vi "Actor Core.vi"(8 "error in":errorcluster, 11 "uService Template in":refnum<class "Common GUI v3.lvclass">) -> (0 "error out":errorcluster, 3 "Actor out":refnum<class "Actor.lvclass">)   [LabVIEW 2026, in "TALOS.lvlib" / "Common GUI v3.lvlib" / "Common GUI v3.lvclass"]
doc: "(<B>Filename</B>: Actor Framework.lvlib:Actor.lvclass:Actor Core.vi)\n\nReceives messages to the actor, reacts to them, and initiates any error handling that may shut the actor down.\n\nDescendant classes may override this VI to append parallel tasks for the actor to complete while it handles messages. Overrides use the Call Parent Class Method node."
uses:
  Common GUI v3.lvclass
  C:/LabVIEW Code/TALOS/builds/Actor Framework PPL/Actor Framework.lvlibp/1abvi3w/vi.lib/ActorFramework/Actor/Actor.lvclass
  C:/LabVIEW Code/TALOS/talos/Father of all uServices/Father of all uServices/Father of all uServices.lvclass
  builds/Actor Framework PPL/Actor Framework.lvlibp/1abvi3w/vi.lib/ActorFramework/Actor/Actor.lvclass
  Common GUI v3.lvclass/Common GUI v3.ctl
  Classes/uService List/uService List.lvclass/uService List.ctl
  Ancestor/Ancestor/Ancestor.lvclass/Ancestor.ctl
  Guardian/Guardian/Buttons_UI.ctl
  Guardian/Guardian Messages/Button Pressed Msg/Button Pressed Msg.lvclass/Button Pressed Msg.ctl
  Remote uService GUI.ctl
  Common GUI v3 Consumer Case Selector.ctl
  Father of all uServices/Father of all uServices Messages/Consumer Msg/Consumer Msg.lvclass/Consumer Msg.ctl
  builds/Actor Framework PPL/Actor Framework.lvlibp/1abvi3w/vi.lib/ActorFramework/Message Enqueuer/Message Priority.ctl
  Ancestor/Ancestor Messages/Process EH Error Msg/Process EH Error Msg.lvclass/Process EH Error Msg.ctl
  Classes/uService List/Get VI Ref.vi
  Classes/uService List/Get Remote GUI.vi
  Classes/uService List/Get Remote Window VI Ref.vi
  Classes/uService List/Get all IDs.vi
  Classes/uService List/Get Properties.vi
  Support VIs/Generate Error.vi
  Father of all uServices/Father of all uServices Messages/Consumer Msg/Send Consumer.vi
  FGV/Error Memory/Get Error Description.vi
  Support VIs/Get PC name.vi
  Ancestor/Ancestor/Read ID.vi
  Support VIs/Get Class Name.vi
  FGV/Error Memory/Error Memory Core.vi
  <vilib>/AdvancedString/Delimited String to 1D String Array.vi
  <vilib>/AdvancedString/Delimited String to 1D String Array (string).vi
  Support VIs/Circus Root Path.vi
  FGV/Error Memory/Error Crt Lvl checker.vi
  FGV/Error Memory/Error Memory Core.vi/40c8088d-b597-4017-91af-faa98e00292e.vi
  FGV/Error Memory/Error Memory Core.vi/d4a3ab98-063c-4e44-b43d-fbdcfe6c2be2.vi
  Father of all uServices/Father of all uServices/Father of all uServices.lvclass
  Support VIs/Global Memory.vi
  <vilib>/Utility/LVClass/Get LV Class Name.vi
  Support VIs/Is in Packed Library.vi
  Support VIs/TALOS Root path.vi
  Support VIs/Read CSV worksheet.vi
  Support VIs/Global Constants.vi
  <vilib>/Utility/error.llb/General Error Handler.vi
  Support VIs/Error Log.vi
  builds/Actor Framework PPL/Actor Framework.lvlibp/1abvi3w/vi.lib/ActorFramework/Message Enqueuer/Enqueue.vi
  <userlib>/_OpenG.lib/lvdata/lvdata.llb/Get Strings from Enum__ogtk.vi
  builds/Actor Framework PPL/Actor Framework.lvlibp/1abvi3w/vi.lib/ActorFramework/Message Enqueuer/Message Enqueuer.lvclass
  Ancestor/Ancestor/Ancestor.lvclass
  <vilib>/Comparison/Equal/Equal Functor/Equal Functor.lvclass
  Guardian/Guardian Messages/Button Pressed Msg/Button Pressed Msg.lvclass
  Father of all uServices/Father of all uServices Messages/Consumer Msg/Consumer Msg.lvclass
  Ancestor/Ancestor Messages/Process EH Error Msg/Process EH Error Msg.lvclass
  Guardian/Guardian/Guardian.lvclass
  Classes/uService List/uService List.lvclass
  TALOS.lvlib
  Common GUI v3.lvlib
panel:
  in  "stop":bool
  in  "remote GUI":bool
  out "Circus Logo":picture
  in  "All uS":bool
  out "Errors":i32(listbox)
  out "uServices Online":T1(c390)
  out "Guardians List":T1(c390)
  out "Run Configuration":string
  out "Run Number":u32
  out "Error Details":string
  out "Kasli Log":string
  out "RUN":bool
  in  "uService to show":string(combo)
  out "ABORT":bool
  out "Guardian ID":string
  # "PRESS CTRL TO ARM"
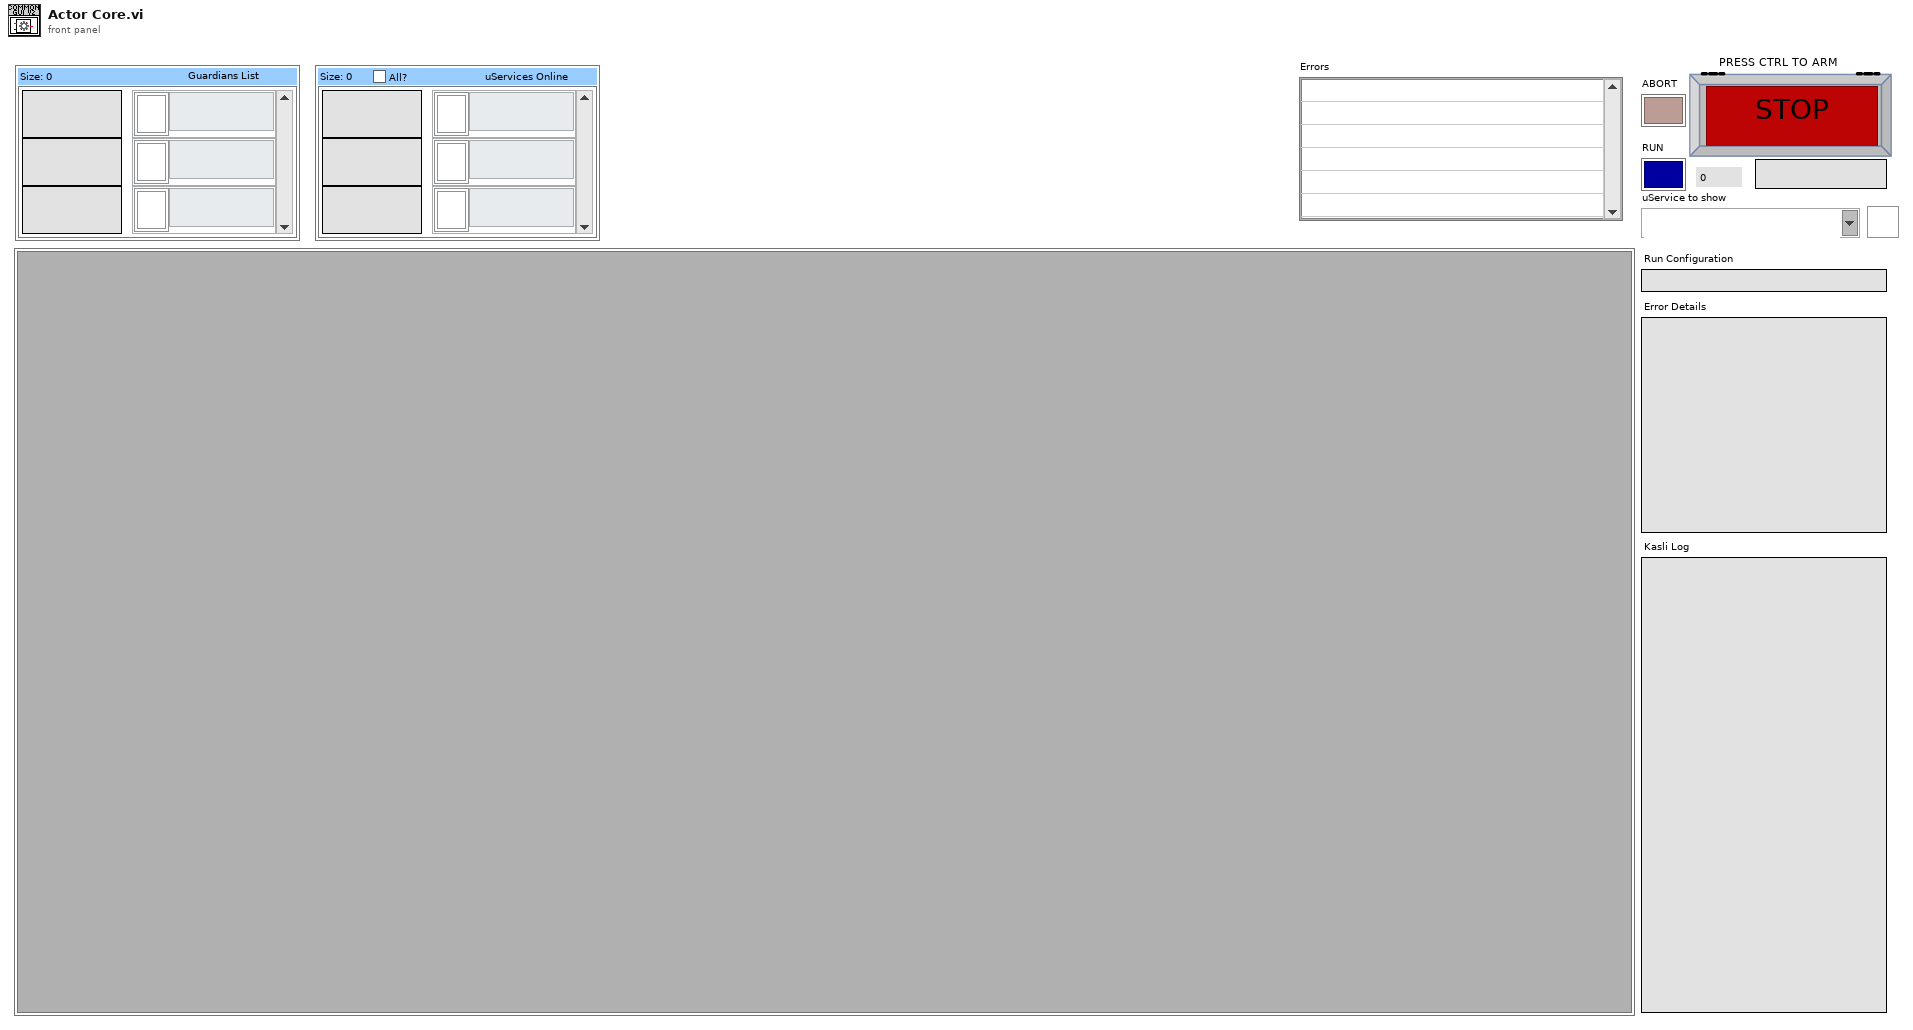
[diagram p1: front panel]
types:
  T1 = map{string, cluster{"Online":bool, "Last Pat":timestamp}}
  T2 = enum16{"None", "On Hover", "On Key Focus", "On Hover or Key Focus"}
  T3 = typedef "TALOS.lvlib/Guardian.lvlib/Guardian.lvclass/Buttons_UI.ctl" = enum16{"Start uService", "Kill uService", "Stop uService", "Stop", "Start online checks", "Stop online checks", "Send Pat to all GDs", "Reload INI files", "Update from GIT", "RUN", "Reset ABORT", "Check Bearer", "Send I Exist", "Change Run Config", "Add uSs from Config", "Realign uSs from Config", "Send Run Config to GD"}
  T4 = typedef "TALOS.lvlib/Common GUI v3.lvlib/Common GUI v3.lvclass/Common GUI v3 Consumer Case Selector.ctl" = enum16{"Update Guardians List", "Update ABORT LED", "Update Guardian ID", "Update Kasli Log", "Update Error Listbox", "Update Run Number", "Change Run LED color", "Update Run Status", "Run Stopped with Errors", "Reset Run LED", "Update Run Config", "Remote GUI"}
  T5 = typedef "TALOS.lvlib/Common GUI v3.lvlib/Remote uService GUI.ctl" = cluster{"Open/Close":bool, "uService ID":string}
  T6 = typedef "Actor Framework.lvlibp/Message Enqueuer.lvclass/Message Priority.ctl" = enum16{"Low", "Normal", "High"}
  T7 = typedef "lveventtype.ctl" = enum32{"Null", "Timeout", "Annotation Menu Selection", "Annotation Menu Selection?", "App Instance Close", "App Instance Close?", "Autoscale Range Change", "Bookmark Info Change", "Cell Edit", "Cell Edit?", "Cursor Grab", "Cursor Grab?", "Cursor Menu Selection", "Cursor Menu Selection?", "Cursor Move", "Cursor Release", "Data Change", "Direction Change", "Display State Change", "Drag Ended", "Drag Enter", "Drag Leave", "Drag Over", "Drag Source Update", "Drag Starting", "Drag Starting?", "Drop", "Exec State Change", "Key Down", "Key Down?", "Key Repeat", "Key Repeat?", "Key Up", "Listbox Double Click", "Menu Activation?", "Menu Selection (App)", "Menu Selection? (App)", "Menu Selection (User)", "Mouse Down", "Mouse Down?", "Mouse Enter", "Mouse Leave", "Mouse Move", "Mouse Up", "Mouse Wheel", "NI Security User Change (App)", "Pane Size", "Panel Close", "Panel Close?", "Panel Resize", "Plot Attribute Change", "Scale Range Change", "Shortcut Menu Activation?", "Shortcut Menu Selection (App)", "Shortcut Menu Selection? (App)", "Shortcut Menu Selection (User)", "Tree Double Click", "Tree Drag", "Tree Drag?", "Tree Drop", "Tree Drop?", "Tree Item Close", "Tree Item Close?", "Tree Item Open", "Tree Item Open?", "URL Change?", "User Event", "Value Change"}
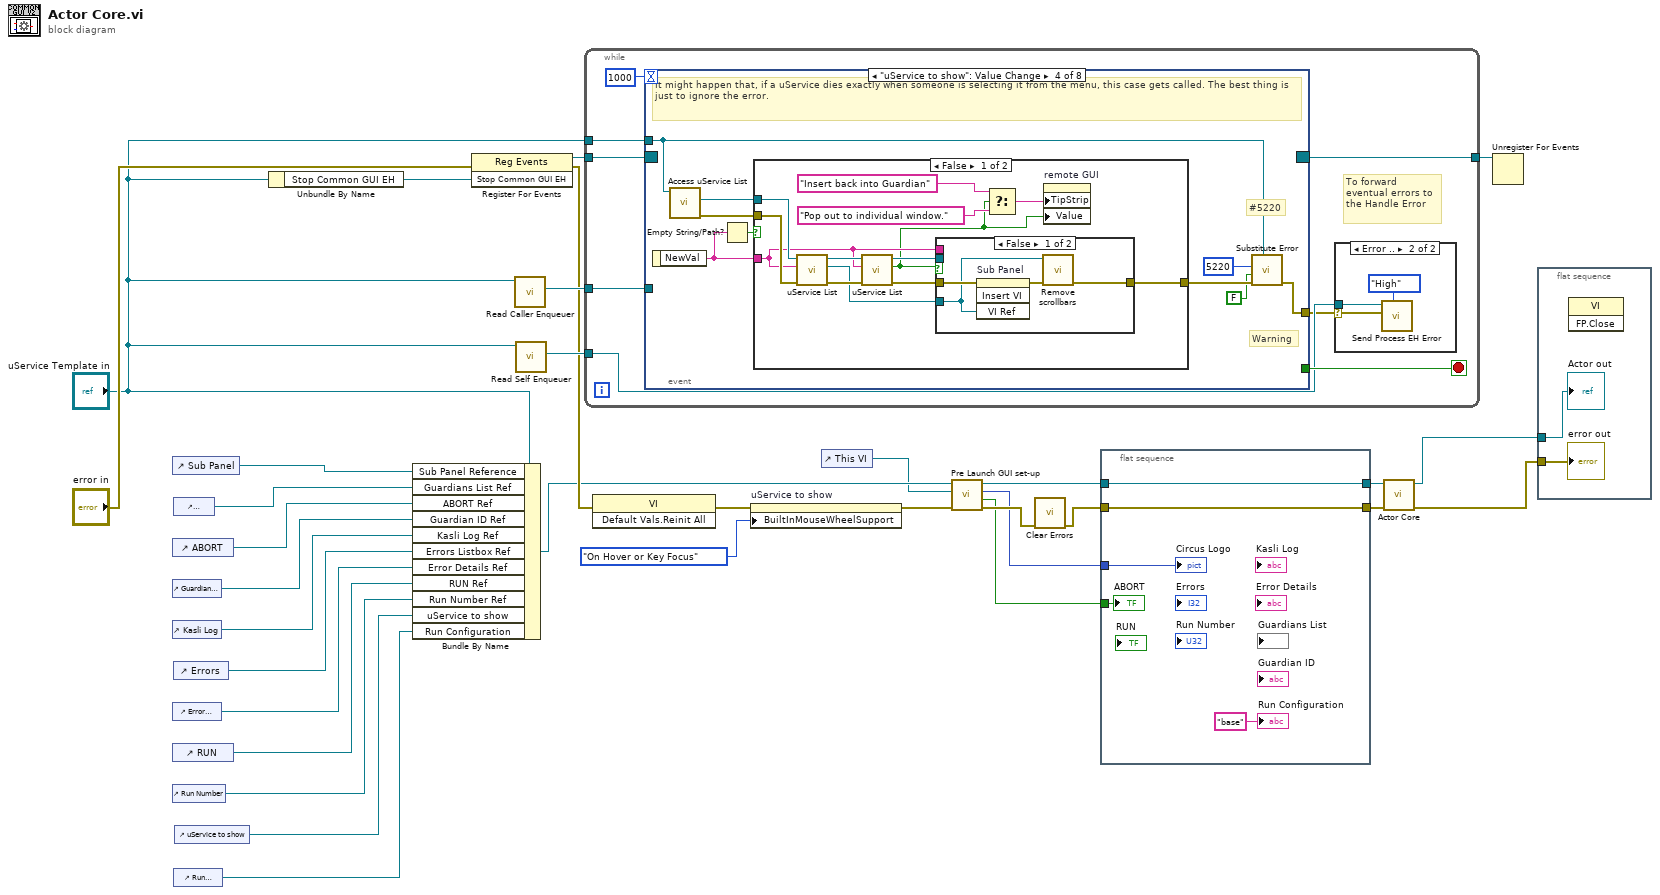
[diagram p0: block diagram]
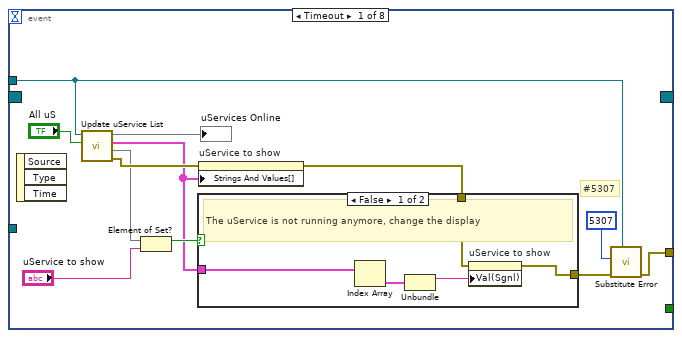
[diagram p2: hidden frame]
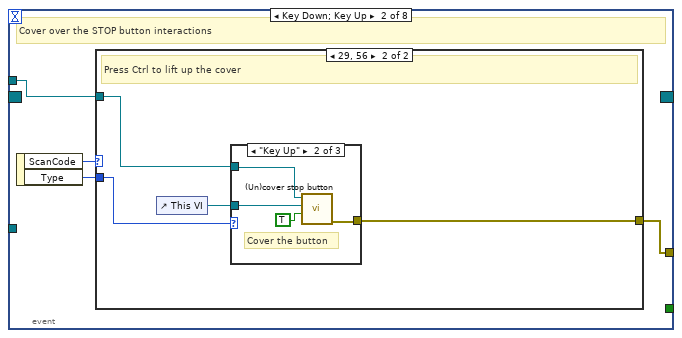
[diagram p4: hidden frame]
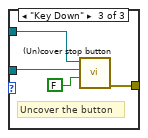
[diagram p7: hidden frame]
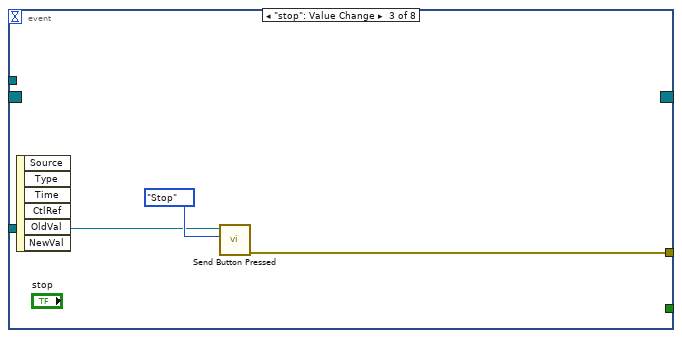
[diagram p8: hidden frame]
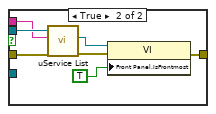
[diagram p9: hidden frame]
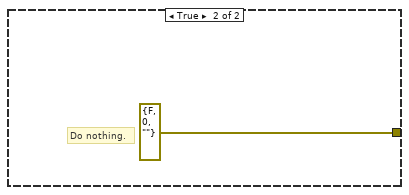
[diagram p10: hidden frame]
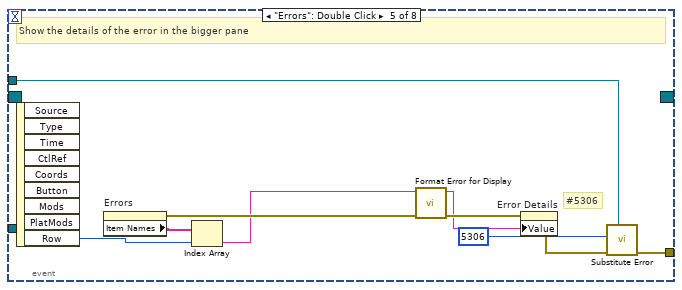
[diagram p11: hidden frame]
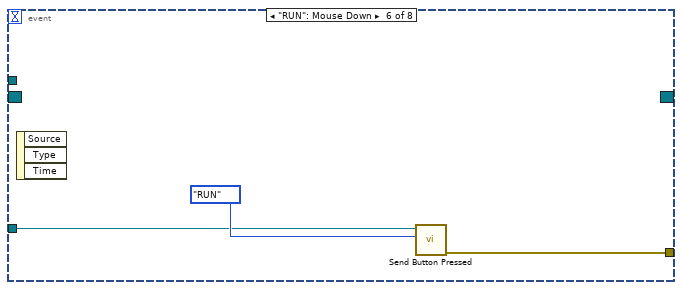
[diagram p12: hidden frame]
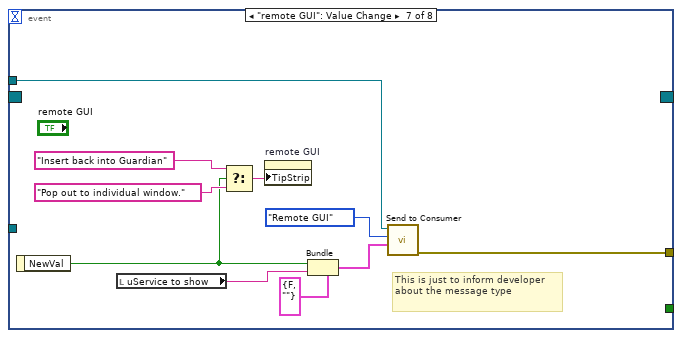
[diagram p13: hidden frame]
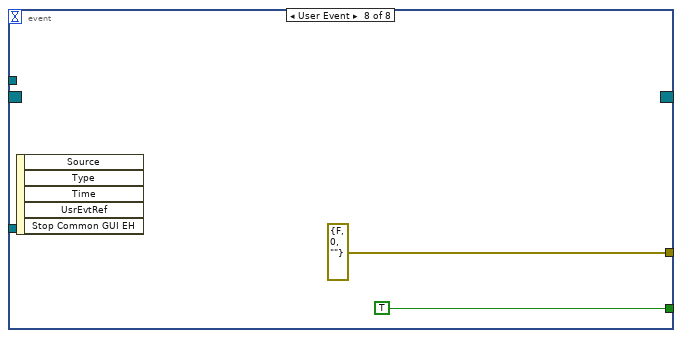
[diagram p14: hidden frame]
diagram:
  n1 = control-ref of="Sub Panel"() -> (w29:refnum<vi>)
  n2 = control-ref of="ABORT"() -> (w22:refnum<vi>)
  n3 = control-ref of="Guardian ID"() -> (w21:refnum<vi>)
  n4 = control-ref of="Kasli Log"() -> (w20:refnum<vi>)
  n5 = control-ref of="Error Details"() -> (w18:refnum<vi>)
  n6 = control-ref of="RUN"() -> (w16:refnum<vi>)
  n7 = control-ref of="Run Number"() -> (w15:refnum<vi>)
  n8 = control-ref of="Guardians List"() -> (w23:refnum<vi>)
  n9 = control-ref of="Errors"() -> (w19:refnum<vi>)
  n10 = control-ref of="Run Configuration"() -> (w5:refnum<vi>)
  n11 = control-ref of="uService to show"() -> (w12:refnum<vi>)
  n12 = Unbundle By Name("uService Template in") -> ("Stop Common GUI EH"=w28:refnum<user-event>)
  n13 = Bundle By Name(cluster="uService Template in", "Sub Panel Reference"=w29, "Guardians List Ref"=w23, "ABORT Ref"=w22, "Guardian ID Ref"=w21, "Kasli Log Ref"=w20, "Errors Listbox Ref"=w19, "Error Details Ref"=w18, "RUN Ref"=w16, "Run Number Ref"=w15, "uService to show"=w12, "Run Configuration"=w5) -> (w11:refnum<class "Common GUI v3.lvclass">)
  n14 = register-events(error in="error in", w28) -> (reference out=w27:refnum<event-registration>, error out=w17:errorcluster)  [unwired: 1 in]
  n15 = call "Read Caller Enqueuer.vi"("Actor"="uService Template in") -> ("Caller Enqueuer"=w25:refnum<class "Message Enqueuer.lvclass">)  [unwired: 10 in]
  n16 = call "Read Self Enqueuer.vi"("Actor"="uService Template in") -> ("Self Enqueuer"=w24:refnum<class "Message Enqueuer.lvclass">)  [unwired: 10 in]
  n17 = while {
    tunnel: w27 -> [w41]
    tunnel: [w39] -> w26
    tunnel: w25 -> [w38]
    tunnel: w24 -> [w36]
    tunnel: "uService Template in" -> [w34]
    stop <- w40 stop-if-true
    # "To forward eventual errors to the Handle Error"
    n18 = event shown="[3] \"uService to show\": Value Change" {
      selector: w41 -> [_ _ _ _ _ _ _ _]
      dyn-events: [_ _ _ _ _ _ _ _] -> w39
      timeout: 1000 -> [_ _ _ _ _ _ _ _]
      tunnel: [_ _ _ _ _ _ _ TRUE] -> w40
      tunnel: w38 -> [_ _ w77 _ _ w124 _ _]
      tunnel: [w45 w60 w76 w84 w119 w123 w132 errorcluster {"status"=FALSE, "code"=0, "source"=""} ("error out")] -> w35
      tunnel: w34 -> [w44 w61 _ w81 w118 _ w131 _]
      event Timeout {
        # "#5307"
        n19 = event-data() -> ()  [unwired: 1 in, 3 out]
        n20 = call "Update uService List.vi"("All uS?"="All uS", "Common GUI v3 in"=w44) -> ("error out"=w53:errorcluster, "Check currently displayed"=w51:set{string}, "For ComboBox"=w48:cluster{"ID":string, "ID":string}[], "Map"=→"uServices Online":map{string, cluster{bool, "Last Pat":timestamp}})  [unwired: 5 in, 1 out]
        n21 = Element of Set?(10:"uService to show", 11:w51) -> (3:w49:bool)
        n22 = property on="uService to show" class="CmbBox"(error in=w53, "Strings And Values[]"=w48) -> (error out=w47:errorcluster)  [unwired: 1 in, 1 out]
        n23 = case shown="False" w49 {
          tunnel: w48 -> [w58 _]
          tunnel: w47 -> [w55 w59]
          tunnel: [w54 w59] -> w46
          frame False {
            # "The uService is not running anymore, change the display"
            n24 = Index Array(array=w58) -> (element=w57:cluster{"ID":string, "ID":string})  [unwired: 1 in]
            n25 = Unbundle(w57) -> ("ID"=w56:string)  [unwired: 1 out]
            n26 = property on="uService to show" class="CmbBox"(error in=w55, "Val(Sgnl)"=w56) -> (error out=w54:errorcluster)  [unwired: 1 in, 1 out]
          }
          frame True {
            # "It's still present, OK"
          }
        }
        n27 = call "Substitute Error.vi"("LabVIEW Object"=w44, "error in (no error)"=w46, "Error Code"=5307) -> ("error out"=w45:errorcluster)  [unwired: 8 in]
      }
      event Key Down; Key Up {
        # "Cover over the STOP button interactions"
        n28 = event-data() -> ("ScanCode"=w63:i16, "Type"=w62:T7)  [unwired: 1 in]
        n29 = case shown="29, 56" w63 {
          tunnel: w62 -> [_ w67]
          tunnel: w61 -> [_ w65]
          tunnel: [_ w64] -> w60
          frame Default {
            # "Any other button, do nothing"
          }
          frame 29, 56 {
            # "Press Ctrl to lift up the cover"
            n30 = control-ref of="This VI"() -> (w66:refnum<vi>)
            n31 = case shown="\"Key Up\"" w67 {
              tunnel: [_ w68 w75] -> w64
              tunnel: w66 -> [_ w70 w73]
              tunnel: w65 -> [_ w69 w72]
              frame "Null", Default {
              }
              frame "Key Up" {
                # "Cover the button"
                n32 = call-dynamic "(Un)cover stop button.vi"("Cover/Uncover"=TRUE, "GUI ref in"=w70, "Common GUI v3 in"=w69) -> ("error out"=w68:errorcluster)  [unwired: 6 in, 2 out]
              }
              frame "Key Down" {
                # "Uncover the button"
                n33 = call-dynamic "(Un)cover stop button.vi"("Cover/Uncover"=FALSE, "GUI ref in"=w73, "Common GUI v3 in"=w72) -> ("error out"=w75:errorcluster)  [unwired: 6 in, 2 out]
              }
            }
          }
        }
      }
      event "stop": Value Change {
        n34 = event-data() -> ()  [unwired: 1 in, 6 out]
        n35 = call "Send Button Pressed.vi"("Button"=Buttons_UI."Stop", "Message Enqueuer"=w77) -> ("error out"=w76:errorcluster)  [unwired: 8 in, 1 out]
      }
      event "uService to show": Value Change {
        # "Warning"
        # "#5220"
        # "It might happen that, if a uService dies exactly when someone is selecting it from the menu, this case gets called. The best thing is just to ignore the error."
        n36 = event-data() -> ("NewVal"=w87:string)  [unwired: 1 in]
        n37 = call-dynamic "Access uService List.vi"("Ancestor in"=w81) -> ("error out"=w80:errorcluster, "uService List out"=w79:refnum<class "uService List.lvclass">)  [unwired: 8 in, 1 out]
        n38 = Empty String/Path?(string/path=w87) -> (empty?=w86:bool)
        n39 = case shown="False" w86 {
          tunnel: [w98 errorcluster {"status"=FALSE, "code"=0, "source"=""} ("error out")] -> w85
          tunnel: w87 -> [w92 _]
          tunnel: w80 -> [w100 _]
          tunnel: w79 -> [w99 _]
          frame False {
            n40 = call-poly "uService List.vi"("error in (no error)"=w100, "ID"=w92, "uService List in"=w99) -> ("error out"=w97:errorcluster, "Vi Ref"=w93:refnum<vi>, "uService List out"=w96:refnum<class "uService List.lvclass">)  [unwired: 6 in]
            n41 = call-poly "uService List.vi"("error in (no error)"=w97, "ID"=w92, "uService List in"=w96) -> ("error out"=w95:errorcluster, "Remote GUI"=w88:bool, "uService List out"=w94:refnum<class "uService List.lvclass">)  [unwired: 6 in]
            n42 = case shown="False" w88 {
              tunnel: [w101 w109] -> w98
              tunnel: w95 -> [w104 w111]
              tunnel: w94 -> [_ w110]
              tunnel: w93 -> [w102 _]
              tunnel: w92 -> [_ w105]
              frame False {
                n43 = invoke on="Sub Panel" class="SubPnl" method="Insert VI"(error in=w104, "VI Ref"=w102) -> (error out=w103:errorcluster)  [unwired: 2 in, 3 out]
                n44 = call "Remove scrollbars.vi"("error in (no error)"=w103, "VI in"=w102) -> ("error out"=w101:errorcluster)  [unwired: 9 in]
              }
              frame True {
                n45 = call-poly "uService List.vi"("error in (no error)"=w111, "ID"=w105, "uService List in"=w110) -> ("error out"=w107:errorcluster, "Vi Ref"=w108:refnum<vi>)  [unwired: 6 in, 1 out]
                n46 = property class="VI"(reference=w108, error in=w107, "Front Panel.IsFrontmost"=TRUE ("Front Panel Window:Is Frontmost")) -> (error out=w109:errorcluster)  [unwired: 1 out]
              }
            }
            n47 = Select(t="Insert back into Guardian", s=w88, f="Pop out to individual window.") -> (s? t:f=w89:string)
            n48 = property on="remote GUI" class="Bool (strict)"("TipStrip"=w89, "Value"=w88) -> ()  [unwired: 2 in, 2 out]
          }
          frame True {
            # "Do nothing."
          }
        }
        n49 = call "Substitute Error.vi"("LabVIEW Object"=w81, "error in (no error)"=w85, "Error/Warning"=FALSE, "Error Code"=5220) -> ("error out"=w84:errorcluster)  [unwired: 7 in]
      }
      event "Errors": Double Click {
        # "#5306"
        # "Show the details of the error in the bigger pane"
        n50 = event-data() -> ("Row"=w121:i32)  [unwired: 1 in, 8 out]
        n51 = property on="Errors" class="LstBox (strict)"() -> (error out=w116:errorcluster, "Item Names"=w122:string[])  [unwired: 2 in, 1 out]
        n52 = Index Array(array=w122, index=w121) -> (element=w114:string)
        n53 = call "Format Error for Display.vi"("error in (no error)"=w116, "Error from Listbox"=w114) -> ("error out"=w115:errorcluster, "Error formatted"=w113:string)  [unwired: 8 in]
        n54 = property on="Error Details" class="Str"(error in=w115, "Value"=w113) -> (error out=w120:errorcluster)  [unwired: 1 in, 1 out]
        n55 = call "Substitute Error.vi"("LabVIEW Object"=w118, "error in (no error)"=w120, "Error Code"=5306) -> ("error out"=w119:errorcluster)  [unwired: 8 in]
      }
      event "RUN": Mouse Down {
        n56 = event-data() -> ()  [unwired: 1 in, 3 out]
        n57 = call "Send Button Pressed.vi"("Button"=Buttons_UI."RUN", "Message Enqueuer"=w124) -> ("error out"=w123:errorcluster)  [unwired: 8 in, 1 out]
      }
      event "remote GUI": Value Change {
        # "This is just to inform developer about the message type"
        n58 = event-data() -> ("NewVal"=w127:bool)  [unwired: 1 in]
        n59 = local read "uService to show"() -> (w134:string)
        n60 = Select(t="Insert back into Guardian", s=w127, f="Pop out to individual window.") -> (s? t:f=w126:string)
        n61 = property on="remote GUI" class="Bool (strict)"("TipStrip"=w126) -> ()  [unwired: 2 in, 2 out]
        n62 = Bundle(cluster=T5 {"Open/Close"=FALSE, "uService ID"=""} ("uService ID"), "Open/Close"=w127, "uService ID"=w134) -> (w133:T5)
        n63 = call "Send to Consumer.vi"("Data"=w133, "Case ID"=Common_GUI_v3_Consumer_Case_Selector."Remote GUI" ("Template Internal v3 Consumer Case Selector"), "uService Template in"=w131) -> ("error out"=w132:errorcluster)  [unwired: 7 in, 1 out]
      }
      event User Event {
        n64 = event-data() -> ()  [unwired: 1 in, 5 out]
      }
    }
    n65 = case shown="Error .." w35 {
      selector: w35 -> [_ w140]
      tunnel: w36 -> [_ w139]
      frame No Error {
      }
      frame Error {
        n66 = call "Send Process EH Error.vi"("Message Priority (Normal)"=Message_Priority."High", "Error to process"=w140, "Message Enqueuer"=w139) -> ()  [unwired: 7 in, 2 out]
      }
    }
  }
  n67 = invoke class="VI" method="Default Vals.Reinit All"(error in=w17) -> (error out=w14:errorcluster)  [unwired: 2 in, 2 out]
  n68 = property on="uService to show" class="CmbBox"(error in=w14, "BuiltInMouseWheelSupport"=T2."On Hover or Key Focus" ("Built-In Mouse Wheel Support")) -> (error out=w9:errorcluster)  [unwired: 1 in, 1 out]
  n69 = control-ref of="This VI"() -> (w10:refnum<vi>)
  n70 = call-dynamic "Pre Launch GUI set-up.vi"("error in (no error)"=w9, "GUI ref"=w10, "Common GUI v3 in"=w11) -> ("error out"=w8:errorcluster, "ABORT?"=w6:bool, "Circus Logo"=w7:picture, "Common GUI v3 out"=w4:refnum<class "Common GUI v3.lvclass">)  [unwired: 5 in]
  n71 = call <vilib>:"Clear Errors.vi"("error in (no error)"=w8) -> ("error out"=w2:errorcluster)  [unwired: 5 in, 1 out]
  n72 = flat-sequence {
    tunnel: w7 -> [w145]
    tunnel: w6 -> [w144]
    tunnel: w4 -> [w143]
    tunnel: [w143] -> w3
    tunnel: w2 -> [w142]
    tunnel: [w142] -> w1
    frame #0 {
      "ABORT" <- w144
      "Circus Logo" <- w145
      "Run Configuration" <- "base" ("Run Configuration")
    }
  }
  n73 = call-parent "Actor Core.vi"("error in"=w1, "uService Template in"=w3) -> ("error out"=w32:errorcluster, "Actor out"=w30:refnum<class "Actor.lvclass">)  [unwired: 8 in]
  n74 = Unregister For Events(event registration refnum=w26) -> ()  [unwired: 1 in, 1 out]
  n75 = flat-sequence {
    tunnel: w32 -> [w147]
    tunnel: w30 -> [w146]
    frame #0 {
      n76 = invoke class="VI" method="FP.Close"() -> ()  [unwired: 3 in, 3 out]
      "error out" <- w147
      "Actor out" <- w146
    }
  }
